vi "Set LVClass Control Label.vi"(8 "error in (no error)":errorcluster, 10 "Name":string, 11 "VI in":refnum<vi>) -> (0 "error out":errorcluster, 3 "VI out":refnum<vi>)   [LabVIEW 2019, in "gRPC Template Creation Utility.lvlib"]
uses:
  <vilib>/Utility/traverseref.llb/TRef TravTarget.ctl
  gRPC Template Creation Utility.lvlib
  <vilib>/Utility/traverseref.llb/VI Scripting - Traverse.lvlib
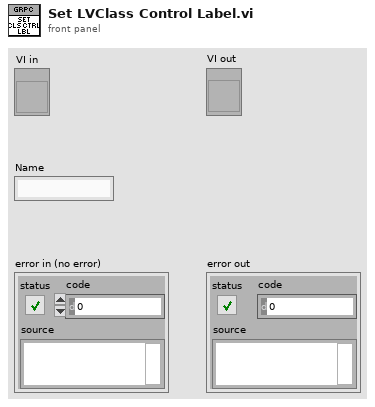
[diagram p1: front panel]
types:
  T1 = typedef "TRef TravTarget.ctl" = enum16{"FP", "BD", "Other"}
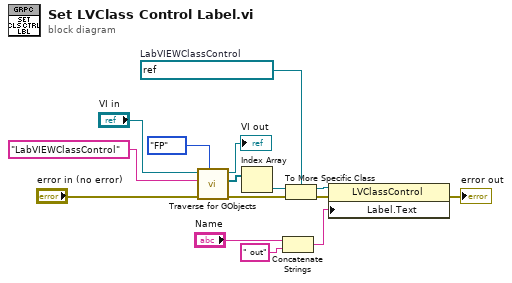
[diagram p0: block diagram]
diagram:
  w7 = refnum<vi> refnum  # LabVIEWClassControl
  n1 = call <vilib>:"Traverse for GObjects.vi"("Traverse Target"=TRef_TravTarget."FP", "error in (no error)"="error in (no error)", "Class Name"="LabVIEWClassControl", "VI Refnum"="VI in") -> ("error out"=w13:errorcluster, "References"=w5:refnum<vi>[], "dup VI Refnum"=→"VI out":refnum<vi>)  [unwired: 4 in, 1 out]
  n2 = Index Array(array=w5) -> (element=w6:refnum<vi>)  [unwired: 1 in]
  n3 = Concatenate Strings("Name", " out" ("string")) -> (w11:string)
  n4 = To More Specific Class(target class=w7, reference=w6, error in=w13) -> (specific class reference=w8:refnum<vi>, error out=w14:errorcluster)
  n5 = property class="LVClassControl"(reference=w8, error in=w14, "Label.Text"=w11) -> (error out=→"error out":errorcluster)  [unwired: 1 out]
